vi "Overview of DVR Qs.vi"() -> ()   [LabVIEW 2021, in "DVR Qs.lvlib"]
uses:
  DVR Qs.lvlib
panel:
  in  "Numeric Control":i32
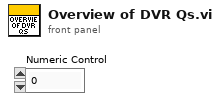
[diagram p1: front panel]
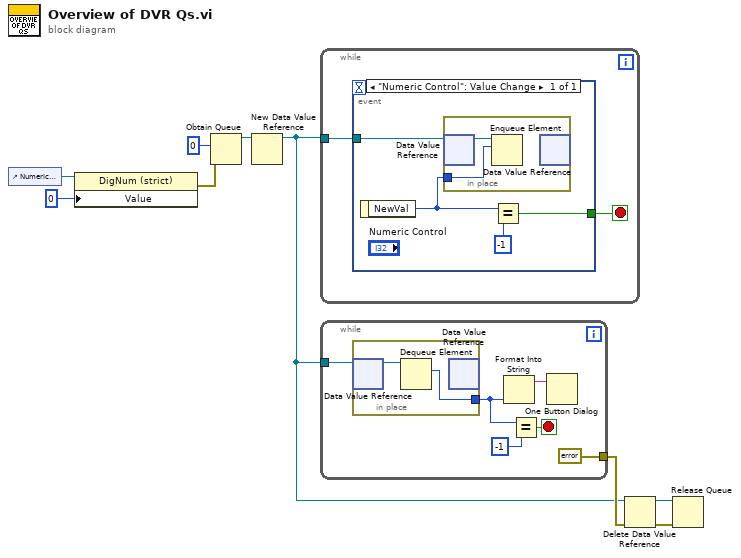
[diagram p0: block diagram]
diagram:
  n1 = control-ref of="Numeric Control"() -> (w9:refnum<vi>)
  n2 = property class="DigNum (strict)"(reference=w9, "Value"=0) -> (error out=w8:errorcluster)  [unwired: 1 in, 1 out]
  n3 = Obtain Queue(element data type=0 ("Value"), error in (no error)=w8) -> (queue out=w5:refnum<queue>)  [unwired: 3 in, 2 out]
  n4 = New Data Value Reference(data value=w5) -> (data value reference=w1:refnum<data-value>)  [unwired: 1 in, 1 out]
  n5 = while {
    tunnel: w1 -> [w10]
    stop <- w11 stop-if-true
    n6 = event shown="[0] \"Numeric Control\": Value Change" {
      selector: _ -> [_]
      dyn-events: _ -> [_]
      timeout: _ -> [_]
      tunnel: w10 -> [w13]
      tunnel: [w14] -> w11
      event "Numeric Control": Value Change {
        n7 = event-data() -> ("NewVal"=w12:i32)  [unwired: 1 in]
        n8 = in-place {
          in-place-border: w12 -> [w16]
          n9 = in-place-dvr #1(w13) -> (w17:refnum<queue>)  [unwired: 1 out]
          n10 = Enqueue Element(queue=w17, element=w16) -> ()  [unwired: 2 in, 3 out]
          n11 = in-place-dvr #1() -> ()  [unwired: 1 in, 2 out]
        }
        n12 = Equal?(x=w12, y=-1) -> (x = y?=w14:bool)
      }
    }
  }
  n13 = while {
    tunnel: w1 -> [w19]
    tunnel: [errorcluster {"status"=FALSE, "code"=0, "source"=""} ("error in (no error)")] -> w3
    stop <- w23 stop-if-true
    n14 = in-place {
      in-place-border: [w24] -> w18
      n15 = in-place-dvr #2(w19) -> (w25:refnum<queue>)  [unwired: 1 out]
      n16 = Dequeue Element(queue=w25) -> (element=w24:i32)  [unwired: 2 in, 3 out]
      n17 = in-place-dvr #2() -> ()  [unwired: 1 in, 2 out]
    }
    n18 = Format Into String(w18) -> (resulting string=w20:string)  [unwired: 3 in, 1 out]
    n19 = Equal?(x=w18, y=-1) -> (x = y?=w23:bool)
    n20 = One Button Dialog(message=w20) -> ()  [unwired: 1 in, 1 out]
  }
  n21 = Delete Data Value Reference(data value reference=w1, error in=w3) -> (data value=w4:refnum<queue>, error out=w2:errorcluster)
  n22 = Release Queue(queue=w4, error in (no error)=w2) -> ()  [unwired: 1 in, 3 out]
